vi "BoolCmd_Recv_Internal.vi"(11 "Command Name":string) -> (0 "error out":errorcluster, 2 "Newest Value":bool, 3 "New Request":bool)   [LabVIEW 2019, in "Trajectory_Library.lvlib"]
uses:
  Trajectory_Library.lvlib
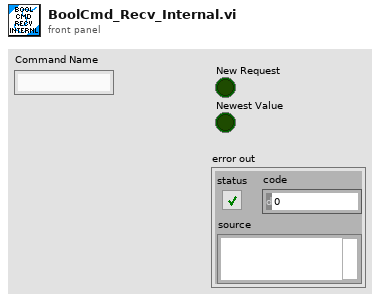
[diagram p1: front panel]
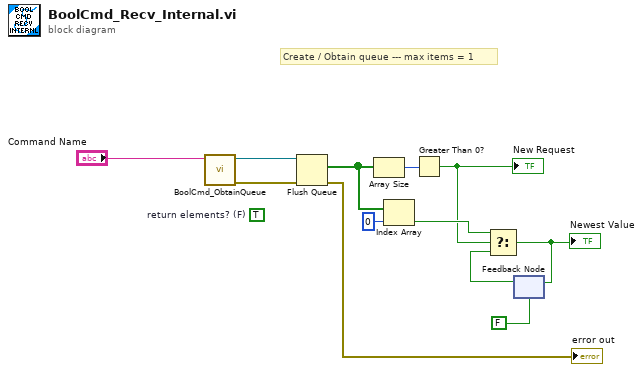
[diagram p0: block diagram]
diagram:
  (unwired) TRUE  # return elements? (F)
  # "Create / Obtain queue --- max items = 1"
  n1 = call "BoolCmd_ObtainQueue.vi"("Command Name"="Command Name") -> ("error out"=w4:errorcluster, "Queue out"=w5:refnum<queue>)  [unwired: 9 in]
  n2 = Flush Queue(queue=w5, error in (no error)=w4) -> (remaining elements=w3:bool[], error out=→"error out":errorcluster)  [unwired: 1 out]
  n3 = Array Size(array=w3) -> (size(s)=w2:i32)
  n4 = Index Array(array=w3, index=0) -> (element=w9:bool)
  n5 = Greater Than 0?(x=w2) -> (x > 0?=w8:bool)
  "New Request" <- w8
  n6 = feedback #1(FALSE) -> (w7:bool)
  n7 = Select(t=w9, s=w8, f=w7) -> (s? t:f=w6:bool)
  "Newest Value" <- w6
  n8 = feedback-in #1(w6) -> ()
